vi "label_integrals.vi"(3 "error in":errorcluster, 4 "Integrals":dbl[](array[numeric]), 5 "Plan":string) -> (0 "error out":errorcluster, 2 "Labelled Integrals":T1(array[cluster]))   [LabVIEW 2020]
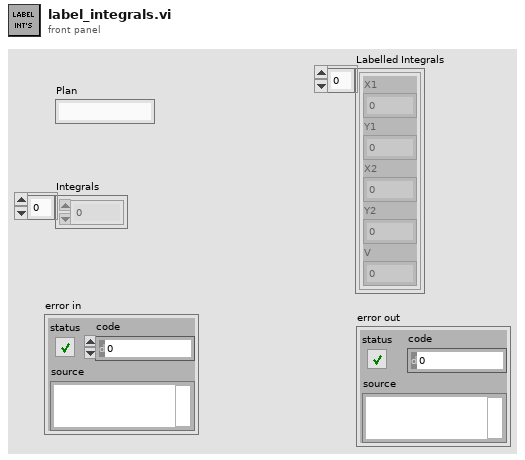
[diagram p1: front panel]
types:
  T1 = cluster{"X1":dbl, "Y1":dbl, "X2":dbl, "Y2":dbl, "V":dbl}[]
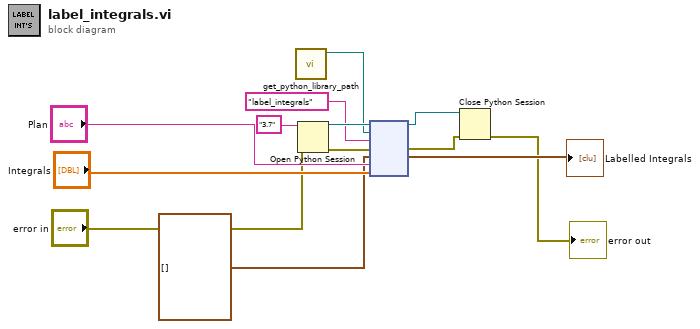
[diagram p0: block diagram]
diagram:
  n1 = call "get_python_library_path.vi"() -> ("Python library path"=w1:path)  [unwired: 11 in]
  n2 = Open Python Session(python version="3.7" ("Python version"), 3:"error in") -> (session out=w11:refnum<k35>, error out=w9:errorcluster)  [unwired: 1 in]
  n3 = node(w11, w1, "label_integrals" ("function name"), w9, T1 [] ("array of clusters"), "Plan", "Integrals") -> (w7:refnum<k35>, w6:errorcluster, →"Labelled Integrals":T1)  [unwired: 2 in, 2 out]
  n4 = Close Python Session(session in=w7, error in=w6) -> (11:→"error out":errorcluster)
